vi "ACP Fetch.vi"(0 "RFmx Handle In":refnum<k21>, 1 "Selector String":string, 5 "Num Carrier Channels":i32, 11 "error in (no error)":errorcluster) -> (4 "RFmx Handle Out":refnum<k21>, 6 "ACP Results":T1 {"Total Carrier Power (dBm or dBm/Hz)" format="%.2f"; "Spectrum (dBm or dBm/Hz)"."y" min=0 max=127 format="%.2f"; "Spectrum (dBm or dBm/Hz)"."dx" format="%^.2e"; "Spectrum (dBm or dBm/Hz)"."x0" format="%^.2e"}, 15 "error out":errorcluster)   [LabVIEW 2016, in "RFmxSpecAn.lvlib"]
uses:
  RFmxSpecAn.lvlib
  Typedefs/ACP Results.ctl
  RFmxNR/Typedefs/NR ACP Offset Results.ctl
  Typedefs/ACP Offset Results.ctl
  Typedefs/ACP Component Carrier Results.ctl
  <vilib>/RFmx/SpecAn/mx/RFmxSpecAn.llb/RFmxSpecAn Build Signal String.vi
  <vilib>/RFmx/RFInstr/mx/RFmxInstr.llb/RFmxInstr Build Signal String.vi
  <vilib>/RFmx/SpecAn/mx/RFmxSpecAn.llb/RFmxSpecAn ACP Fetch Offset Measurement (Array).vi
  <vilib>/RFmx/SpecAn/mx/RFmxSpecAn.llb/RFmxSpecAn ACP Fetch Carrier Measurement.vi
  <vilib>/RFmx/SpecAn/mx/RFmxSpecAn.llb/RFmxSpecAn ACP Fetch Total Carrier Power.vi
  <vilib>/RFmx/SpecAn/mx/RFmxSpecAn.llb/RFmxSpecAn ACP Fetch Spectrum.vi
  <resource>/objmgr/RFmxSpecAn.rc
  RFmxNR/RFmxNR.lvlib
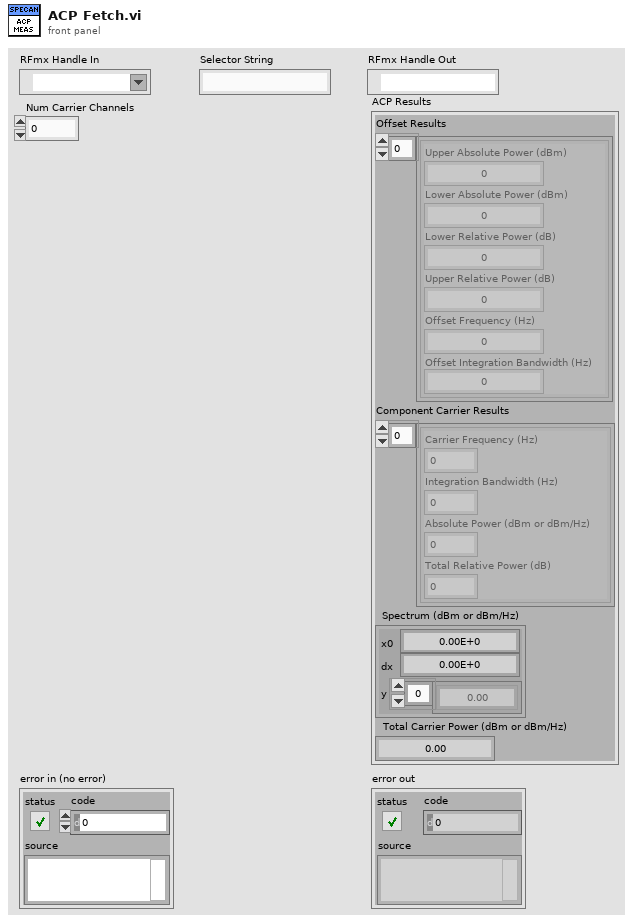
[diagram p1: front panel]
types:
  T1 = typedef "RFmxSpecAn.lvlib/ACP Results.ctl" = cluster{"Offset Results":T2[], "Component Carrier Results":cluster{"Carrier Frequency (Hz)":dbl, "Integration Bandwidth (Hz)":dbl, "Absolute Power (dBm or dBm/Hz)":dbl, "Total Relative Power (dB)":dbl}[], "Spectrum (dBm or dBm/Hz)":cluster{"x0":dbl, "dx":dbl, "y":sgl[]}, "Total Carrier Power (dBm or dBm/Hz)":dbl}
  T2 = typedef "RFmxNR.lvlib/NR ACP Offset Results.ctl" = cluster{"Upper Absolute Power (dBm)":dbl, "Lower Absolute Power (dBm)":dbl, "Lower Relative Power (dB)":dbl, "Upper Relative Power (dB)":dbl, "Offset Frequency (Hz)":dbl, "Offset Integration Bandwidth (Hz)":dbl}
  T3 = typedef "RFmxSpecAn.lvlib/ACP Offset Results.ctl" = cluster{"Lower Absolute Power (dBm)":dbl, "Upper Absolute Power (dBm)":dbl, "Lower Relative Power (dB)":dbl, "Upper Relative Power (dB)":dbl, "Offset Frequency (Hz)":dbl, "Offset Integration Bandwidth (Hz)":dbl}
  T4 = typedef "RFmxSpecAn.lvlib/ACP Component Carrier Results.ctl" = cluster{"Carrier Frequency (Hz)":dbl, "Integration Bandwidth (Hz)":dbl, "Absolute Power (dBm or dBm/Hz)":dbl, "Total Relative Power (dB)":dbl}
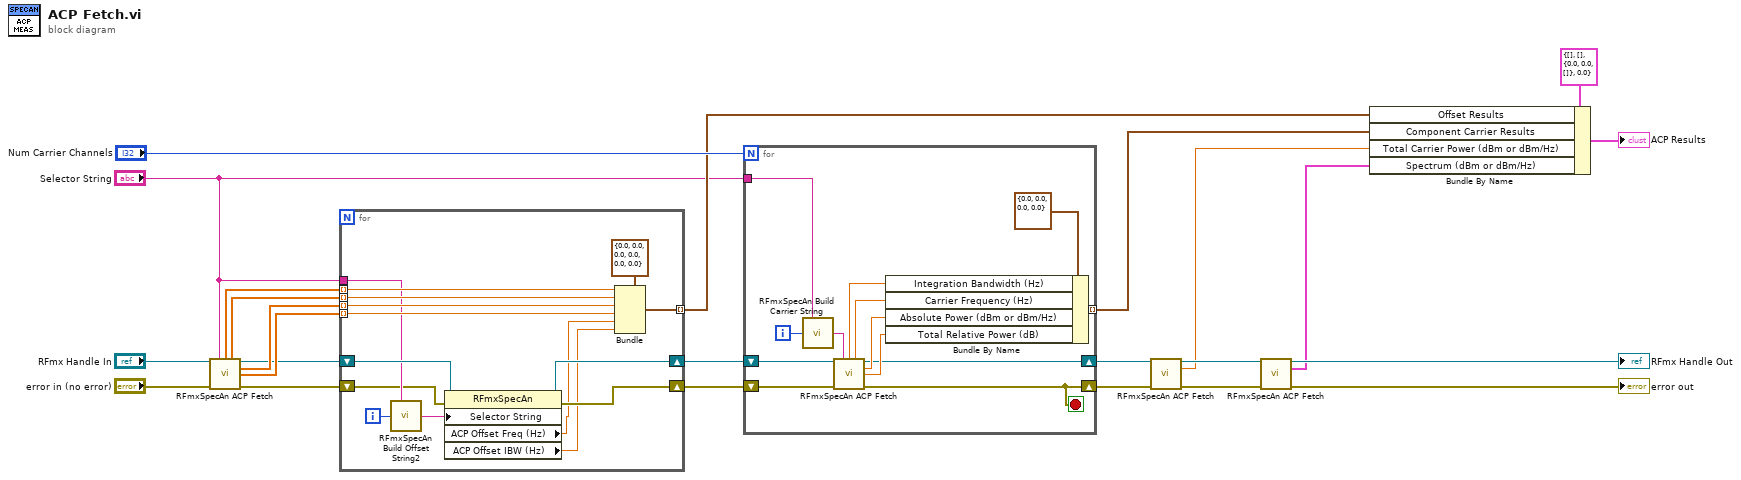
[diagram p0: block diagram]
diagram:
  n1 = call-poly <vilib>:"RFmxSpecAn ACP Fetch.vi"("Instrument Handle In"="RFmx Handle In", "Selector String"="Selector String", "error in (no error)"="error in (no error)") -> ("Lower Absolute Power (dBm or dBm/Hz)"=w15:dbl[], "Upper Absolute Power (dBm or dBm/Hz)"=w14:dbl[], "Instrument Handle Out"=w10:refnum<k21>, "Lower Relative Power (dB)"=w13:dbl[], "Upper Relative Power (dB)"=w12:dbl[], "error out"=w11:errorcluster)  [unwired: 7 in]
  n2 = for {
    shift-right: [w38] -> w6
    shift-left: w10 -> [w36]
    shift-right: [w39] -> w5
    shift-left: w11 -> [w25]
    tunnel: [w37] -> w7 mode=indexing
    tunnel: w15 -> [w35] mode=indexing
    tunnel: w14 -> [w34] mode=indexing
    tunnel: w13 -> [w33] mode=indexing
    tunnel: w12 -> [w32] mode=indexing
    tunnel: "Selector String" -> [w30]
    i -> [w29]
    n3 = call <vilib>:"RFmxSpecAn Build Offset String2.vi"("Selector String"=w30, "Offset Number"=w29) -> ("Selector String Out"=w26:string)  [unwired: 13 in]
    n4 = property class="RFmxSpecAn"(reference=w36, error in=w25, "Selector String"=w26) -> (reference out=w38:refnum<k21>, error out=w39:errorcluster, "ACP Offset Freq (Hz)"=w27:dbl, "ACP Offset IBW (Hz)"=w28:dbl)
    n5 = Bundle(cluster=T3 {"Lower Absolute Power (dBm)"=0.0, "Upper Absolute Power (dBm)"=0.0, "Lower Relative Power (dB)"=0.0, "Upper Relative Power (dB)"=0.0, "Offset Frequency (Hz)"=0.0, "Offset Integration Bandwidth (Hz)"=0.0} ("ACP Offset Results"), "Lower Absolute Power (dBm)"=w35, "Upper Absolute Power (dBm)"=w34, "Lower Relative Power (dB)"=w33, "Upper Relative Power (dB)"=w32, "Offset Frequency (Hz)"=w27, "Offset Integration Bandwidth (Hz)"=w28) -> (w37:T3)
  }
  n6 = for {
    N: "Num Carrier Channels" -> [_]
    shift-right: [w46] -> w24
    shift-left: w6 -> [w52]
    shift-right: [w44] -> w23
    shift-left: w5 -> [w51]
    tunnel: [w47] -> w3 mode=indexing
    tunnel: "Selector String" -> [w42]
    i -> [w41]
    stop <- w44 stop-if-true
    n7 = call <vilib>:"RFmxSpecAn Build Carrier String.vi"("Signal Name"=w42, "Carrier Number"=w41) -> ("Carrier String"=w43:string)  [unwired: 13 in]
    n8 = call-poly <vilib>:"RFmxSpecAn ACP Fetch.vi"("Instrument Handle In"=w52, "Selector String"=w43, "error in (no error)"=w51) -> ("Integration Bandwidth (Hz)"=w45:dbl, "Frequency (Hz)"=w50:dbl, "Instrument Handle Out"=w46:refnum<k21>, "Absolute Power (dBm or dBm/Hz)"=w49:dbl, "Total Relative Power (dB)"=w48:dbl, "error out"=w44:errorcluster)  [unwired: 7 in]
    n9 = Bundle By Name(cluster=T4 {"Carrier Frequency (Hz)"=0.0, "Integration Bandwidth (Hz)"=0.0, "Absolute Power (dBm or dBm/Hz)"=0.0, "Total Relative Power (dB)"=0.0} ("ACP Component Carrier Results"), "Integration Bandwidth (Hz)"=w45, "Carrier Frequency (Hz)"=w50, "Absolute Power (dBm or dBm/Hz)"=w49, "Total Relative Power (dB)"=w48) -> (w47:T4)
  }
  n10 = call-poly <vilib>:"RFmxSpecAn ACP Fetch.vi"("Instrument Handle In"=w24, "error in (no error)"=w23) -> ("Instrument Handle Out"=w22:refnum<k21>, "Total Carrier Power (dBm or dBm/Hz)"=w2:dbl, "error out"=w21:errorcluster)  [unwired: 11 in]
  n11 = call-poly <vilib>:"RFmxSpecAn ACP Fetch.vi"("Instrument Handle In"=w22, "error in (no error)"=w21) -> ("Instrument Handle Out"=→"RFmx Handle Out":refnum<k21>, "Spectrum (dBm or dBm/Hz)"=w1:cluster{"x0":dbl, "dx":dbl, "y":sgl[]}, "error out"=→"error out":errorcluster)  [unwired: 11 in]
  n12 = Bundle By Name(cluster=T1 {"Offset Results"=[], "Component Carrier Results"=[], "Spectrum (dBm or dBm/Hz)"={"x0"=0.0, "dx"=0.0, "y"=[]}, "Total Carrier Power (dBm or dBm/Hz)"=0.0} ("ACP Results"), "Offset Results"=w7, "Component Carrier Results"=w3, "Total Carrier Power (dBm or dBm/Hz)"=w2, "Spectrum (dBm or dBm/Hz)"=w1) -> (→"ACP Results":T1)
